vi "SrvEventText.vi"(0 "CR_LF":bool, 2 "var_Event":T1, 3 "error in (no error)":errorcluster) -> (7 "EventText":string, 10 "error out":errorcluster)   [LabVIEW 2018, in "Snap7.lvlib"]
uses:
  Snap7.lvlib
  windows/lv_snap7.dll
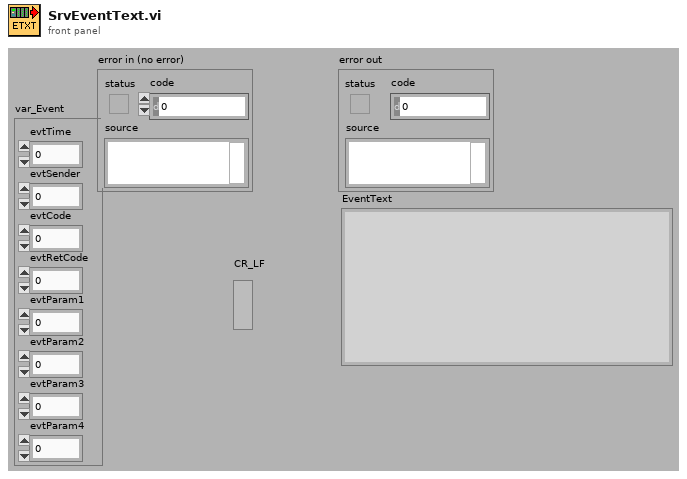
[diagram p1: front panel]
types:
  T1 = cluster{"evtTime":u32, "evtSender":i32, "evtCode":u32, "evtRetCode":u16, "evtParam1":u16, "evtParam2":u16, "evtParam3":u16, "evtParam4":u16}
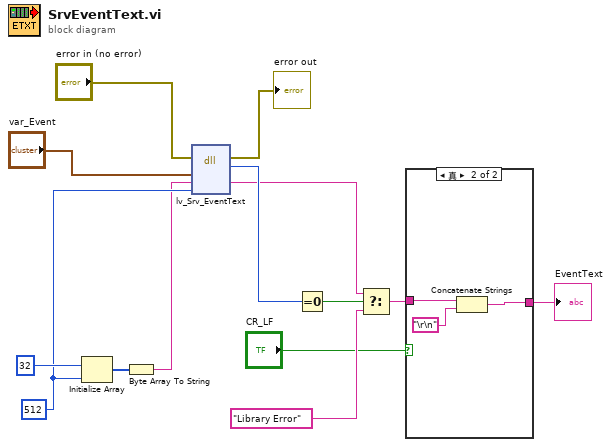
[diagram p0: block diagram]
diagram:
  w10 = 512 ("Dimension Size")
  n1 = Initialize Array(u8 32 ("Element Data"), w10) -> (w12:u8[])
  n2 = Byte Array To String(unsigned byte array=w12) -> (string=w9:string)
  n3 = dll-call lib="C:/Users/WanLiMing/Downloads/snap7-full-1.4.2/snap7-full-1.4.2/LabVIEW/lib/windows/lv_snap7.dll" fn="lv_Srv_EventText"(error in="error in (no error)", "Event"="var_Event", "EventText"=w9, "TextLen"=w10) -> (error out=→"error out":errorcluster, "return type"=w7:i32, "EventText"=w6:string)  [unwired: 4 in, 1 out]
  n4 = Equal To 0?(x=w7) -> (x = 0?=w8:bool)
  n5 = Select(t=w6, s=w8, f="Library Error") -> (s? t:f=w2:string)
  n6 = case shown="真" "CR_LF" {
    tunnel: w2 -> [w15 w18]
    tunnel: [w15 w16] -> w1
    frame False {
    }
    frame True {
      n7 = Concatenate Strings(w18, "\r\n") -> (w16:string)
    }
  }
  "EventText" <- w1
